vi "Main.vi"() -> ()   [LabVIEW 2024, in "Wordle Scorer.lvlib"]
uses:
  Wordle Scorer.lvlib
  Result.ctl
  515452d5-10dc-45b2-bfa0-4ce66a95e6dd.vi
panel:
  out "Inspection Result":string
  out "Folder":path
  in  "Running":bool
  out "Solver VI":path
  in  "Rerun":bool
  out "submission":i32
  in  "Result":T1
  out "Response":string
  out "Upload Debug":string
  in  "Skip":bool
  in  "Upload":bool
  out "Success":bool
  out "Run Time":dbl format="%_6f"
  in  "Cancel":bool
  in  "Run":bool
  out "Download Debug":string
  out "Get Next Debug":string
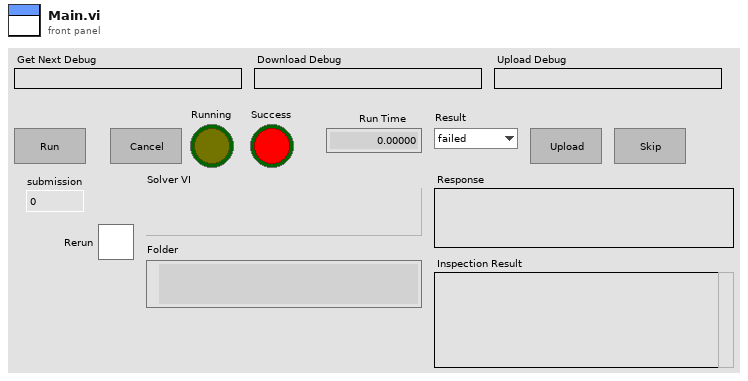
[diagram p1: front panel]
types:
  T1 = typedef "Wordle Scorer.lvlib/Result.ctl" = enum16{"failed", "complete", "error", "timeout", "ineligible"}
  T2 = enum8{"Enabled", "Disabled", "Disabled and Grayed Out"}
  T3 = typedef "Word Search Scorer.lvlib/Solver VI Ref Type.ctl" = refnum<vi>
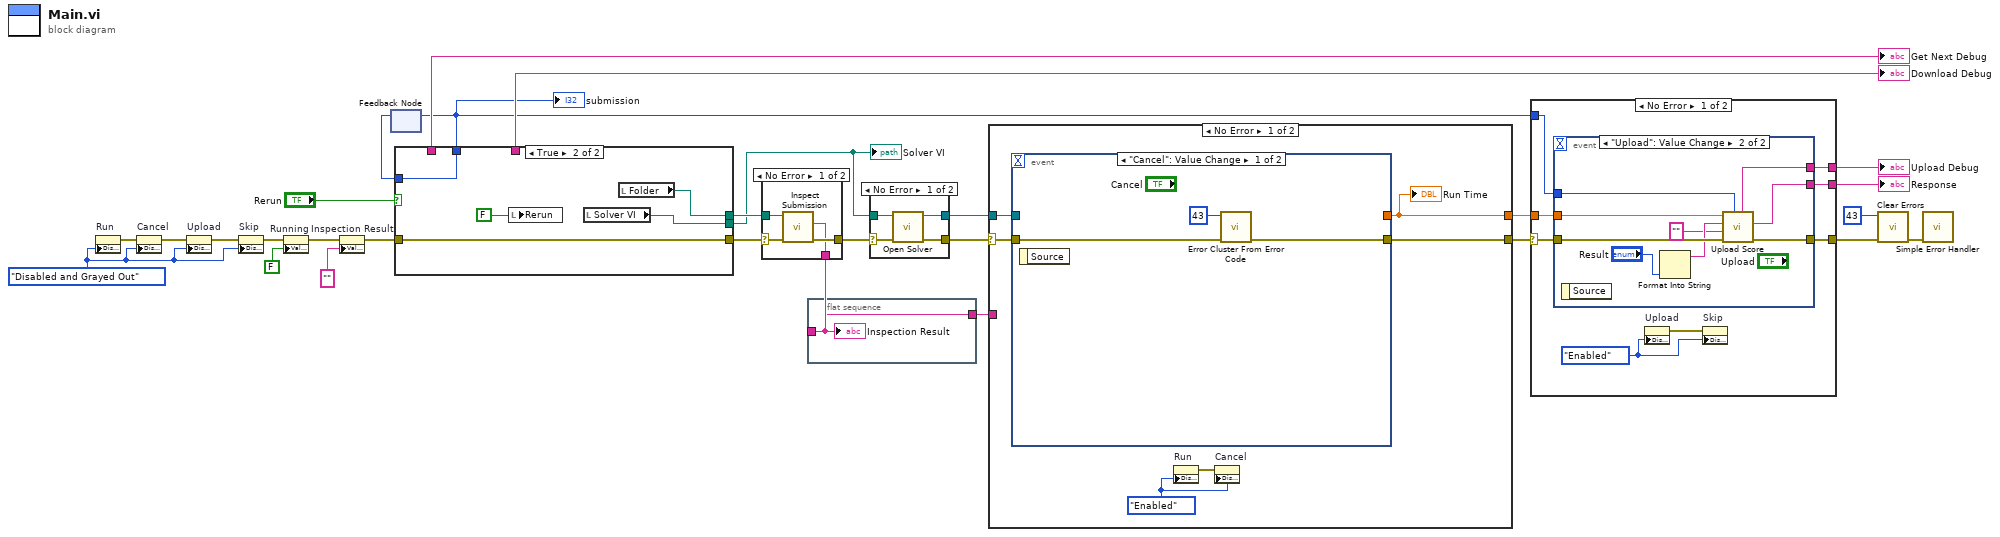
[diagram p0: block diagram]
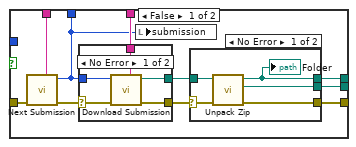
[diagram p3: hidden frame]
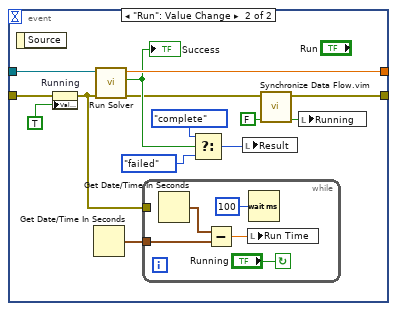
[diagram p7: hidden frame]
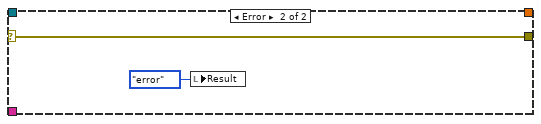
[diagram p8: hidden frame]
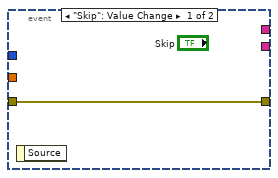
[diagram p9: hidden frame]
diagram:
  w15 = T2."Disabled and Grayed Out" ("Disabled")
  n1 = property on="Run" class="Bool"("DisabledEnum"=w15) -> (error out=w24:errorcluster)  [unwired: 2 in, 1 out]
  n2 = property on="Cancel" class="Bool"(error in=w24, "DisabledEnum"=w15) -> (error out=w23:errorcluster)  [unwired: 1 in, 1 out]
  n3 = property on="Upload" class="Bool"(error in=w23, "DisabledEnum"=w15) -> (error out=w16:errorcluster)  [unwired: 1 in, 1 out]
  n4 = property on="Skip" class="Bool"(error in=w16, "DisabledEnum"=w15) -> (error out=w14:errorcluster)  [unwired: 1 in, 1 out]
  n5 = property on="Running" class="Bool (strict)"(error in=w14, "Value"=FALSE ("Running")) -> (error out=w3:errorcluster)  [unwired: 1 in, 1 out]
  n6 = property on="Inspection Result" class="Str"(error in=w3, "Value"="" ("Inspection Result")) -> (error out=w2:errorcluster)  [unwired: 1 in, 1 out]
  n7 = feedback #1() -> (w11:i32)  [unwired: 1 in]
  n8 = case shown="True" "Rerun" {
    tunnel: [w39 _] -> w29
    tunnel: [w37 _] -> w28
    tunnel: [w31 w56] -> w12
    tunnel: [w34 w55] -> w9
    tunnel: [w33 w53] -> w6
    tunnel: w2 -> [w32 w55]
    tunnel: w11 -> [_ w56]
    tunnel: [w30 w52] -> w8
    frame False {
      n9 = call "Next Submission.vi"("error in (no error)"=w32) -> ("error out"=w38:errorcluster, "submission"=w31:i32, "Profile URL"=w39:string)  [unwired: 8 in]
      n10 = case shown="No Error" w38 {
        selector: w38 -> [w43 w45]
        tunnel: w31 -> [w44 _]
        tunnel: [w42 _] -> w37
        tunnel: [w41 _] -> w35
        tunnel: [w40 w45] -> w36
        frame No Error {
          n11 = call "Download Submission.vi"("error in (no error)"=w43, "submission"=w44) -> ("error out"=w40:errorcluster, "Zip Path"=w41:path, "Profile URL"=w42:string)  [unwired: 7 in]
        }
        frame Error {
        }
      }
      n12 = local write "submission"(w31) -> ()
      n13 = case shown="No Error" w36 {
        selector: w36 -> [w50 w51]
        tunnel: w35 -> [w49 _]
        tunnel: [w48 _] -> w33
        tunnel: [w47 w51] -> w34
        tunnel: [w46 _] -> w30
        frame No Error {
          n14 = call "Unpack Zip.vi"("error in (no error)"=w50, "Zip"=w49) -> ("error out"=w47:errorcluster, "Solver VI"=w48:path, "Folder"=w46:path)  [unwired: 7 in]
          "Folder" <- w46
        }
        frame Error {
        }
      }
    }
    frame True {
      n15 = local write "Rerun"(FALSE ("Rerun")) -> ()
      n16 = local read "Solver VI"() -> (w53:path)
      n17 = local read "Folder"() -> (w52:path)
    }
  }
  "Get Next Debug" <- w29
  "Download Debug" <- w28
  "submission" <- w12
  "Solver VI" <- w6
  n18 = feedback-in #1(w12) -> ()
  n19 = case shown="No Error" w9 {
    selector: w9 -> [w59 w61]
    tunnel: w8 -> [w60 _]
    tunnel: [w58 w61] -> w7
    tunnel: [w57 _] -> w5
    frame No Error {
      n20 = call "Inspect Submission.vi"("error in (no error)"=w59, "Folder"=w60) -> ("error out"=w58:errorcluster, "Inspection Result"=w57:string)  [unwired: 7 in, 1 out]
    }
    frame Error {
    }
  }
  n21 = flat-sequence {
    tunnel: w5 -> [w62]
    tunnel: [w62] -> w4
    frame #0 {
      "Inspection Result" <- w62
    }
  }
  n22 = case shown="No Error" w7 {
    selector: w7 -> [w65 w67]
    tunnel: w6 -> [w66 _]
    tunnel: [w64 _] -> w27
    tunnel: [w63 w67] -> w26
    frame No Error {
      n23 = call "Open Solver.vi"("error in (no error)"=w65, "Solver Path"=w66) -> ("error IO"=w63:errorcluster, "Solver VI"=w64:T3)  [unwired: 8 in]
    }
    frame Error {
    }
  }
  n24 = case shown="No Error" w26 {
    selector: w26 -> [w72 w97]
    tunnel: w27 -> [w73 _]
    tunnel: [w71 w97] -> w25
    tunnel: [w68 _] -> w19
    tunnel: w4 -> [_ _]
    frame No Error {
      w70 = T2."Enabled" ("Disabled")
      n25 = event shown="[0] \"Cancel\": Value Change" {
        selector: _ -> [_ _]
        dyn-events: _ -> [_ _]
        timeout: _ -> [_ _]
        tunnel: w73 -> [_ w90]
        tunnel: w72 -> [w76 w79]
        tunnel: [w74 w82] -> w71
        tunnel: [_ w89] -> w68
        event "Cancel": Value Change {
          n26 = event-data() -> ()  [unwired: 1 in, 1 out]
          n27 = call <vilib>:"Error Cluster From Error Code.vi"("error in (no error)"=w76, "error code (0)"=43) -> ("error out"=w74:errorcluster)  [unwired: 7 in]
        }
        event "Run": Value Change {
          n28 = event-data() -> ()  [unwired: 1 in, 1 out]
          n29 = property on="Running" class="Bool (strict)"(error in=w79, "Value"=TRUE ("Running")) -> (error out=w77:errorcluster)  [unwired: 1 in, 1 out]
          n30 = Get Date/Time In Seconds() -> (seconds since 1Jan1904=w84:timestamp)
          n31 = call "Run Solver.vi"("error in (no error)"=w77, "Solver VI"=w90) -> ("error out"=w83:errorcluster, "Completed"=w88:bool, "Run Time"=w89:dbl)  [unwired: 7 in]
          "Success" <- w88
          n32 = while {
            tunnel: w84 -> [w94]
            tunnel: w77 -> [_]
            stop <- "Running" continue-if-true
            n33 = Get Date/Time In Seconds() -> (seconds since 1Jan1904=w95:timestamp)
            n34 = Subtract(x=w95, y=w94) -> (x-y=w92:dbl)
            n35 = local write "Run Time"(w92) -> ()
            n36 = Wait (ms)(milliseconds to wait=u32 100) -> ()  [unwired: 1 out]
          }
          n37 = Select(t=Result."complete" ("Result"), s=w88, f=Result."failed" ("Result")) -> (s? t:f=w86:T1)
          n38 = local write "Result"(w86) -> ()
          n39 = call "Synchronize Data Flow.vim"("input 4"=FALSE, "input 1"=w83) -> ("output 4"=w80:bool, "output 1"=w82:errorcluster)  [unwired: 2 in, 2 out]
          n40 = local write "Running"(w80) -> ()
        }
      }
      "Run Time" <- w68
      n41 = property on="Run" class="Bool"("DisabledEnum"=w70) -> (error out=w69:errorcluster)  [unwired: 2 in, 1 out]
      n42 = property on="Cancel" class="Bool"(error in=w69, "DisabledEnum"=w70) -> ()  [unwired: 1 in, 2 out]
    }
    frame Error {
      n43 = local write "Result"(Result."error" ("Result")) -> ()
    }
  }
  n44 = case shown="No Error" w25 {
    selector: w25 -> [w105 w116]
    tunnel: [w104 w116] -> w22
    tunnel: w19 -> [w103 _]
    tunnel: w12 -> [w102 _]
    tunnel: [w101 _] -> w18
    tunnel: [w100 _] -> w17
    frame No Error {
      w98 = T2."Enabled" ("Disabled")
      n45 = event shown="[1] \"Upload\": Value Change" {
        selector: _ -> [_ _]
        dyn-events: _ -> [_ _]
        timeout: _ -> [_ _]
        tunnel: w105 -> [w106 w115]
        tunnel: [w106 w113] -> w104
        tunnel: w103 -> [_ w114]
        tunnel: w102 -> [_ w109]
        tunnel: [_ w112] -> w101
        tunnel: [_ w111] -> w100
        event "Skip": Value Change {
          n46 = event-data() -> ()  [unwired: 1 in, 1 out]
        }
        event "Upload": Value Change {
          n47 = event-data() -> ()  [unwired: 1 in, 1 out]
          n48 = Format Into String("Result") -> (resulting string=w108:string)  [unwired: 3 in, 1 out]
          n49 = call "Upload Score.vi"("submission"=w109, "error in (no error)"=w115, "result"="", "status"=w108, "Run Time"=w114) -> ("error out"=w113:errorcluster, "Response"=w111:string, "Profile URL"=w112:string)  [unwired: 4 in]
        }
      }
      n50 = property on="Upload" class="Bool"("DisabledEnum"=w98) -> (error out=w99:errorcluster)  [unwired: 2 in, 1 out]
      n51 = property on="Skip" class="Bool"(error in=w99, "DisabledEnum"=w98) -> ()  [unwired: 1 in, 2 out]
    }
    frame Error {
    }
  }
  "Upload Debug" <- w18
  "Response" <- w17
  n52 = call <vilib>:"Clear Errors.vi"("error in (no error)"=w22, "specific error code to clear (0: all)"=43) -> ("error out"=w21:errorcluster)  [unwired: 4 in, 1 out]
  n53 = call <vilib>:"Simple Error Handler.vi"("error in (no error)"=w21) -> ()  [unwired: 4 in, 5 out]
